vi "ActorPool.vi"(6 "Functions":T1=enum."GetAll", 8 "ErrorIn":errorcluster, 9 "ActorRef":refnum<vi>, 10 "GuiRef":refnum<vi>) -> (0 "ErrorOut":errorcluster, 2 "AllActorRefs":refnum<vi>[](array[refnum]), 3 "AllGuiRefs":refnum<vi>[](array[refnum]))   [LabVIEW 2021, in "YActor.lvclass"]
uses:
  YActor.lvclass
  private/ActorPoolFunctions.ctl
  YActor.lvclass/YActor.ctl
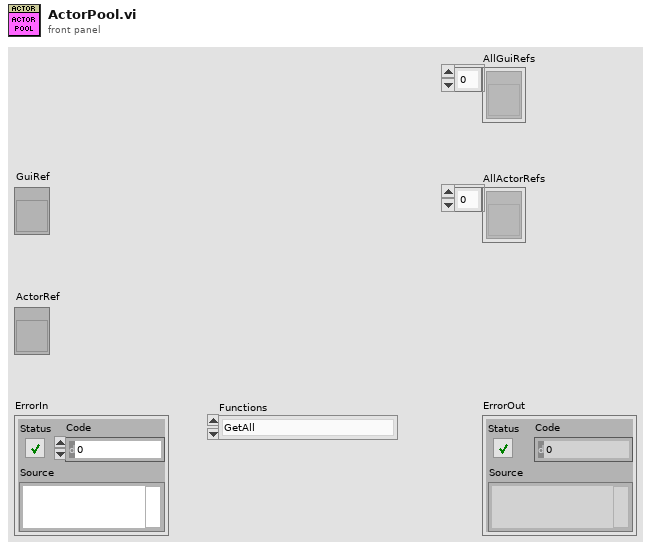
[diagram p1: front panel]
types:
  T1 = typedef "YActor.lvclass/ActorPoolFunctions.ctl" = enum16{"Add", "GetAll", "Delete"}
  T2 = enum32{"Bad", "Idle", "Run top level", "Running"}
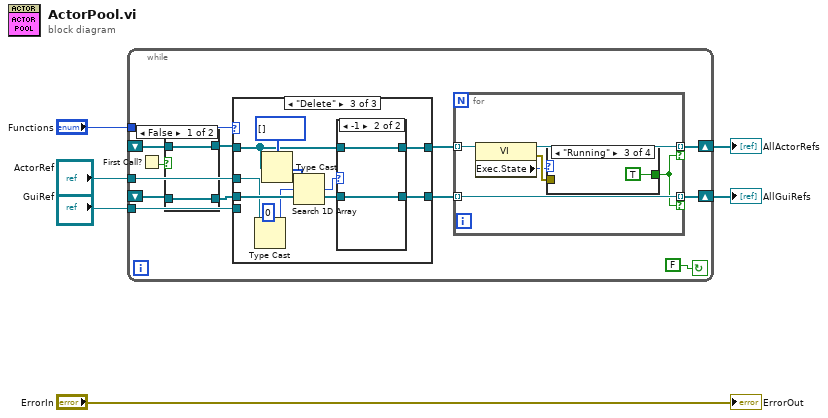
[diagram p0: block diagram]
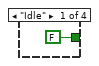
[diagram p3: hidden frame]
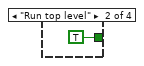
[diagram p4: hidden frame]
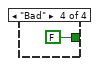
[diagram p5: hidden frame]
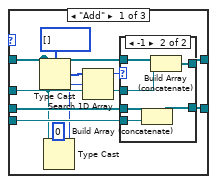
[diagram p6: hidden frame]
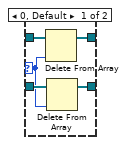
[diagram p9: hidden frame]
diagram:
  n1 = while {
    tunnel: "Functions" -> [w19]
    shift-right: [w16] -> w3
    shift-left: _ -> [w10]
    tunnel: "ActorRef" -> [w17]
    shift-right: [w14] -> w1
    shift-left: _ -> [w8]
    tunnel: "GuiRef" -> [w13]
    stop <- FALSE continue-if-true
    n2 = First Call?() -> (First Call?: T/F=w11:bool)
    n3 = case shown="False" w11 {
      tunnel: [w21 _] -> w9
      tunnel: w10 -> [w21 _]
      tunnel: w8 -> [w20 _]
      tunnel: [w20 _] -> w7
      frame False {
      }
      frame True {
      }
    }
    n4 = case shown="\"Delete\"" w19 {
      tunnel: w9 -> [w38 w52 w55]
      tunnel: [w42 w52 w62] -> w12
      tunnel: w17 -> [w37 _ w54]
      tunnel: w7 -> [w41 w51 w60]
      tunnel: [w39 w51 w61] -> w15
      tunnel: w13 -> [w40 _ _]
      frame "Add" {
        n5 = Type Cast(type=i32[] [], x=w38) -> (*(type *) &x=w34:i32[])
        n6 = Type Cast(type=0, x=w37) -> (*(type *) &x=w33:i32)
        n7 = Search 1D Array(1D array=w34, element=w33) -> (index of element=w32:i32)  [unwired: 1 in]
        n8 = case shown="-1" w32 {
          tunnel: [w44 w50] -> w42
          tunnel: w41 -> [w43 w49]
          tunnel: w40 -> [_ w48]
          tunnel: [w43 w47] -> w39
          tunnel: w38 -> [w44 w46]
          tunnel: w37 -> [_ w45]
          frame 0, Default {
          }
          frame -1 {
            n9 = Build Array (concatenate)(w49, w48) -> (w47:refnum<vi>[])
            n10 = Build Array (concatenate)(w46, w45) -> (w50:refnum<vi>[])
          }
        }
      }
      frame "GetAll" {
      }
      frame "Delete" {
        n11 = Type Cast(type=0, x=w54) -> (*(type *) &x=w56:i32)
        n12 = Type Cast(type=i32[] [], x=w55) -> (*(type *) &x=w57:i32[])
        n13 = Search 1D Array(1D array=w57, element=w56) -> (index of element=w53:i32)  [unwired: 1 in]
        n14 = case shown="-1" w53 {
          selector: w53 -> [w63 _]
          tunnel: [w66 w69] -> w62
          tunnel: w55 -> [w67 w69]
          tunnel: [w65 w68] -> w61
          tunnel: w60 -> [w64 w68]
          frame 0, Default {
            n15 = Delete From Array(array=w67, index=w63) -> (array with subset deleted=w66:refnum<vi>[])  [unwired: 1 in, 1 out]
            n16 = Delete From Array(array=w64, index=w63) -> (array with subset deleted=w65:refnum<vi>[])  [unwired: 1 in, 1 out]
          }
          frame -1 {
          }
        }
      }
    }
    n17 = for {
      tunnel: w12 -> [w26] mode=indexing
      tunnel: [w24] -> w16 mode=indexing if=w22
      tunnel: w15 -> [w25] mode=indexing
      tunnel: [w25] -> w14 mode=indexing if=w22
      n18 = property class="VI"(reference=w26) -> (reference out=w24:refnum<vi>, error out=w27:errorcluster, "Exec.State"=w23:T2)  [unwired: 1 in]
      n19 = case shown="\"Running\"" w23 {
        tunnel: [FALSE TRUE TRUE FALSE] -> w22
        tunnel: w27 -> [_ _ _ _]
        frame "Idle" {
        }
        frame "Run top level" {
        }
        frame "Running" {
        }
        frame "Bad" {
        }
      }
    }
  }
  "AllActorRefs" <- w3
  "AllGuiRefs" <- w1
  "ErrorOut" <- "ErrorIn"
